vi "Copy Image (ARGB with ARGB Mask).vi"(8 "error in (no error)":errorcluster, 9 "ARGB Image Mask in":T1, 10 "ARGB Image Destination in":T1, 11 "ARGB Image Source in":T1) -> (0 "error out":errorcluster, 3 "ARGB Image Destination":T1)   [LabVIEW 2020, in "image.lvlib"]
doc: "Copy pixles where the Mask is non-zero from the Source Image to the Destination Image.\n\nThe Destination Image must be sized to match the Source Image."
uses:
  image.lvlib
  ARGB Image.ctl
  3b1fb24f-4521-4d3d-a8b9-ed3d08148c99.vi
  <vilib>/Utility/error.llb/Error Cluster From Error Code.vi
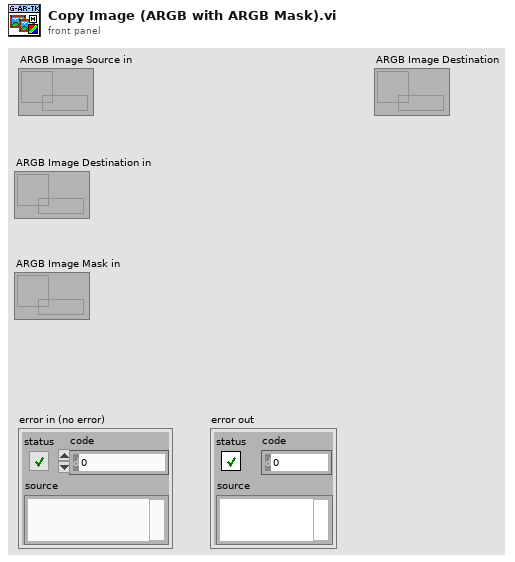
[diagram p1: front panel]
types:
  T1 = typedef "image.lvlib/ARGB Image.ctl" = refnum<data-value>
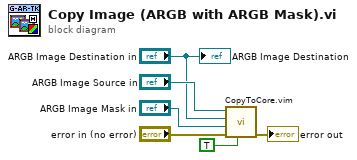
[diagram p0: block diagram]
diagram:
  n1 = call "CopyToCore.vim"("Has Mask"=TRUE, "error in (no error)"="error in (no error)", "Mask"="ARGB Image Mask in", "Dst"="ARGB Image Destination in", "Src"="ARGB Image Source in") -> ("error out"=→"error out":errorcluster)  [unwired: 6 in]
  "ARGB Image Destination" <- "ARGB Image Destination in"
